vi "ValidateVersion.vi"(8 "error in (no error)":errorcluster, 11 "SaveForPrevious in":refnum<class "SaveForPrevious.lvclass">) -> (0 "error out":errorcluster, 3 "SaveForPrevious out":refnum<class "SaveForPrevious.lvclass">)   [LabVIEW 2014, in "SaveForPrevious.lvclass"]
doc: "Ensures the save version is provided."
uses:
  SaveForPrevious.lvclass
  SaveForPrevious.lvclass/SaveForPrevious.ctl
  <nishared>/LabVIEW CLI/Operations/Utilities/OperationErrorType.ctl
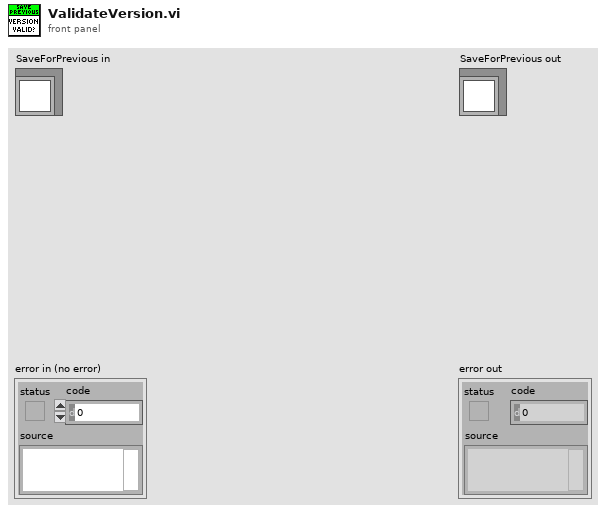
[diagram p1: front panel]
types:
  T1 = typedef "OperationErrorType.ctl" = enum16{"RequiredArgumentMissing", "UnknownArguments", "LoggerSetMultipleTimes", "OperationBrokenError"}
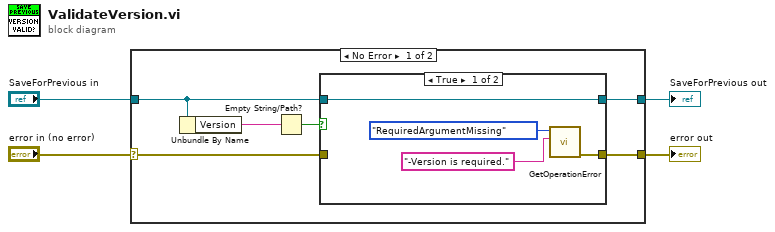
[diagram p0: block diagram]
diagram:
  n1 = case shown="No Error" "error in (no error)" {
    selector: "error in (no error)" -> [w8 w18]
    tunnel: [w7 w18] -> w3
    tunnel: [w5 w17] -> w1
    tunnel: "SaveForPrevious in" -> [w6 w17]
    frame No Error {
      n2 = Unbundle By Name(w6) -> ("Version"=w9:string)
      n3 = Empty String/Path?(string/path=w9) -> (empty?=w10:bool)
      n4 = case shown="True" w10 {
        tunnel: w8 -> [_ w16]
        tunnel: [w13 w16] -> w7
        tunnel: w6 -> [w14 w15]
        tunnel: [w14 w15] -> w5
        frame True {
          n5 = call <nishared>:"GetOperationError.vi"("Additional Information"="-Version is required.", "Operation Error Type"=OperationErrorType."RequiredArgumentMissing") -> ("error out"=w13:errorcluster)  [unwired: 9 in]
        }
        frame False {
        }
      }
    }
    frame Error {
    }
  }
  "error out" <- w3
  "SaveForPrevious out" <- w1
